vi "getErrorDevice.vi"(8 "error in (no error)":errorcluster, 11 "AtomChipHWC in":refnum<class "AtomChipHWC.lvclass">) -> (0 "error out":errorcluster, 2 "Devices":string[](array[string]), 3 "AtomChipHWC out":refnum<class "AtomChipHWC.lvclass">)   [LabVIEW 2011, in "Hardware.lvlib" / "HWControllers.lvlib" / "AtomChipHWC.lvclass"]
uses:
  AtomChipHWC.lvclass
  AtomChipHWC.lvclass/AtomChipHWC.ctl
  HWController.lvclass
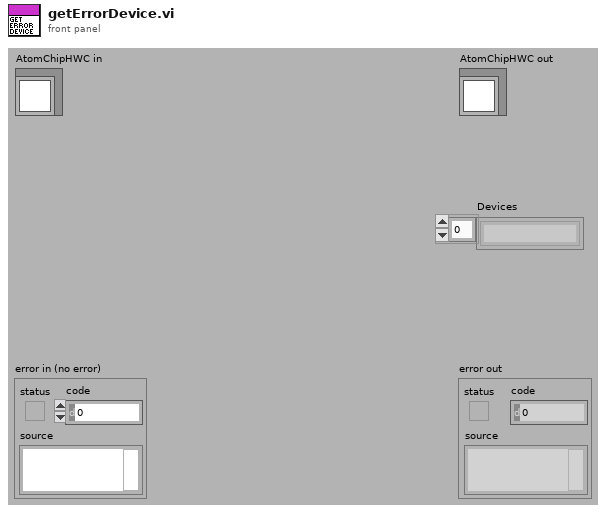
[diagram p1: front panel]
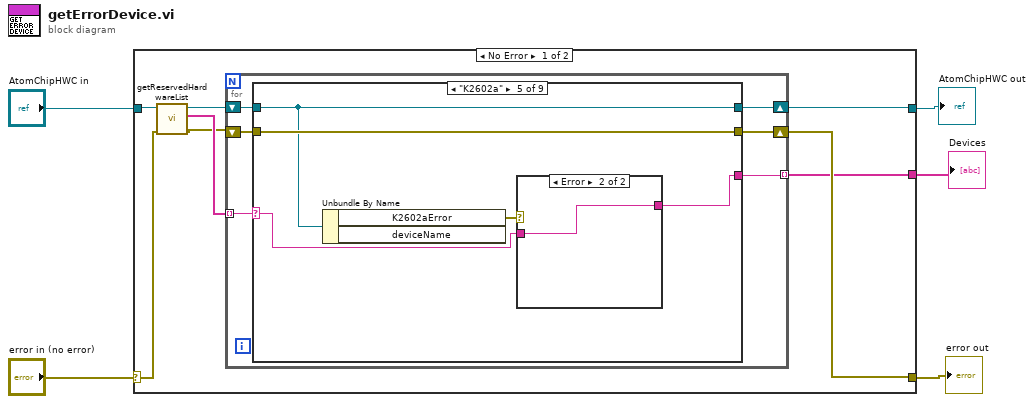
[diagram p0: block diagram]
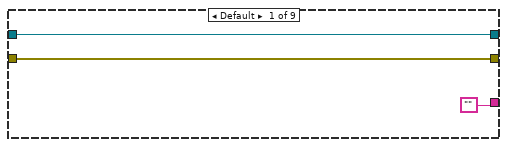
[diagram p2: hidden frame]
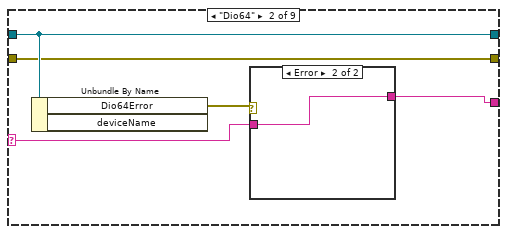
[diagram p3: hidden frame]
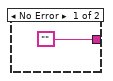
[diagram p4: hidden frame]
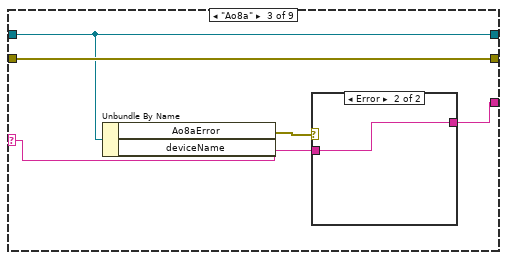
[diagram p5: hidden frame]
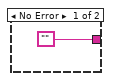
[diagram p6: hidden frame]
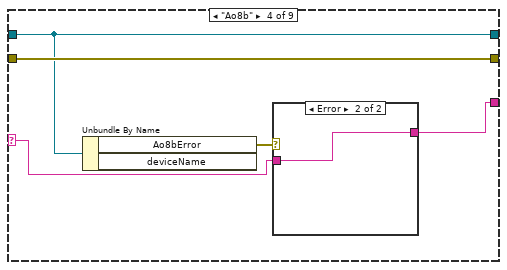
[diagram p7: hidden frame]
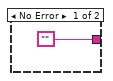
[diagram p8: hidden frame]
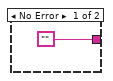
[diagram p9: hidden frame]
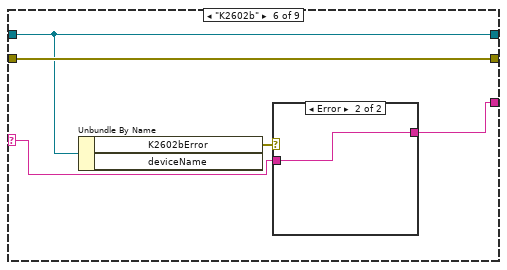
[diagram p10: hidden frame]
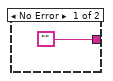
[diagram p11: hidden frame]
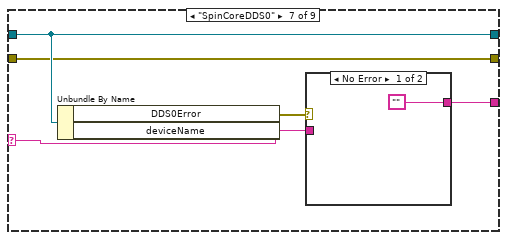
[diagram p12: hidden frame]
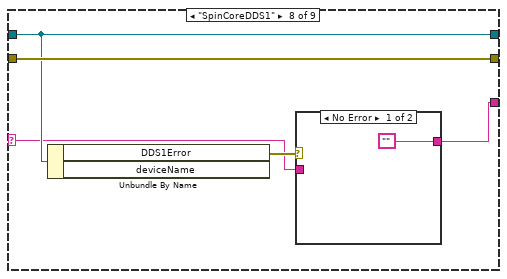
[diagram p14: hidden frame]
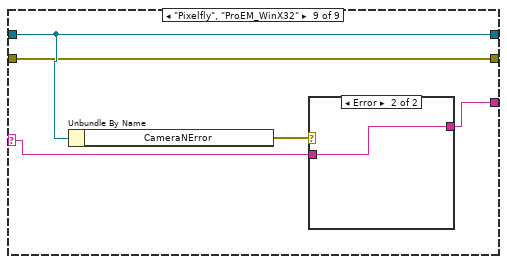
[diagram p16: hidden frame]
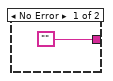
[diagram p17: hidden frame]
diagram:
  n1 = case shown="No Error" "error in (no error)" {
    selector: "error in (no error)" -> [w6 w80]
    tunnel: [w12 w80] -> w4
    tunnel: [w13 w79] -> w2
    tunnel: "AtomChipHWC in" -> [w10 w79]
    tunnel: [w11 _] -> w1
    frame No Error {
      n2 = call "getReservedHardwareList.vi"("error in (no error)"=w6, "HWController.lvclass in"=w10) -> ("error out"=w7:errorcluster, "reservedHardwareList"=w8:string[], "HWController.lvclass out"=w9:refnum<class "AtomChipHWC.lvclass">)  [unwired: 7 in]
      n3 = for {
        shift-right: [w18] -> w13
        shift-left: w9 -> [w19]
        tunnel: w8 -> [w16] mode=indexing
        shift-right: [w15] -> w12
        shift-left: w7 -> [w17]
        tunnel: [w14] -> w11 mode=indexing
        n4 = case shown="\"K2602a\"" w16 {
          selector: w16 -> [_ w23 w30 w37 w44 w51 w58 w65 w72]
          tunnel: w19 -> [w22 w27 w33 w40 w47 w54 w62 w66 w75]
          tunnel: [w22 w27 w33 w40 w47 w54 w62 w66 w75] -> w18
          tunnel: w17 -> [w21 w26 w34 w41 w48 w55 w61 w68 w74]
          tunnel: [w21 w26 w34 w41 w48 w55 w61 w68 w74] -> w15
          tunnel: ["" w24 w31 w38 w45 w52 w59 w67 w73] -> w14
          frame Default {
          }
          frame "Dio64" {
            n5 = Unbundle By Name(w27) -> ("Dio64Error"=w25:errorcluster)  [unwired: 1 out]
            n6 = case shown="Error" w25 {
              tunnel: ["" w29] -> w24
              tunnel: w23 -> [_ w29]
              frame No Error {
              }
              frame Error {
              }
            }
          }
          frame "Ao8a" {
            n7 = Unbundle By Name(w33) -> ("Ao8aError"=w32:errorcluster)  [unwired: 1 out]
            n8 = case shown="Error" w32 {
              tunnel: ["" w36] -> w31
              tunnel: w30 -> [_ w36]
              frame No Error {
              }
              frame Error {
              }
            }
          }
          frame "Ao8b" {
            n9 = Unbundle By Name(w40) -> ("Ao8bError"=w39:errorcluster)  [unwired: 1 out]
            n10 = case shown="Error" w39 {
              tunnel: ["" w43] -> w38
              tunnel: w37 -> [_ w43]
              frame No Error {
              }
              frame Error {
              }
            }
          }
          frame "K2602a" {
            n11 = Unbundle By Name(w47) -> ("K2602aError"=w46:errorcluster)  [unwired: 1 out]
            n12 = case shown="Error" w46 {
              tunnel: ["" w50] -> w45
              tunnel: w44 -> [_ w50]
              frame No Error {
              }
              frame Error {
              }
            }
          }
          frame "K2602b" {
            n13 = Unbundle By Name(w54) -> ("K2602bError"=w53:errorcluster)  [unwired: 1 out]
            n14 = case shown="Error" w53 {
              tunnel: ["" w57] -> w52
              tunnel: w51 -> [_ w57]
              frame No Error {
              }
              frame Error {
              }
            }
          }
          frame "SpinCoreDDS0" {
            n15 = Unbundle By Name(w62) -> ("DDS0Error"=w60:errorcluster)  [unwired: 1 out]
            n16 = case shown="No Error" w60 {
              tunnel: ["" w64] -> w59
              tunnel: w58 -> [_ w64]
              frame No Error {
              }
              frame Error {
              }
            }
          }
          frame "SpinCoreDDS1" {
            n17 = Unbundle By Name(w66) -> ("DDS1Error"=w69:errorcluster)  [unwired: 1 out]
            n18 = case shown="No Error" w69 {
              tunnel: ["" w71] -> w67
              tunnel: w65 -> [_ w71]
              frame No Error {
              }
              frame Error {
              }
            }
          }
          frame "Pixelfly", "ProEM_WinX32" {
            n19 = Unbundle By Name(w75) -> ("CameraNError"=w76:errorcluster)
            n20 = case shown="Error" w76 {
              tunnel: ["" w78] -> w73
              tunnel: w72 -> [_ w78]
              frame No Error {
              }
              frame Error {
              }
            }
          }
        }
      }
    }
    frame Error {
    }
  }
  "error out" <- w4
  "AtomChipHWC out" <- w2
  "Devices" <- w1
